vi "SPD.Overall Progress tracker.vi"(8 "Error In":errorcluster, 9 "Num of temps":i32, 10 "Current temprature index":i32, 11 "Slide in":refnum<vi>) -> (0 "Error Out":errorcluster, 3 "Slide out":refnum<vi>)   [LabVIEW 2018]
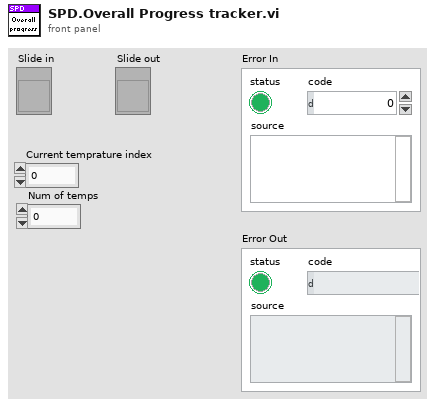
[diagram p1: front panel]
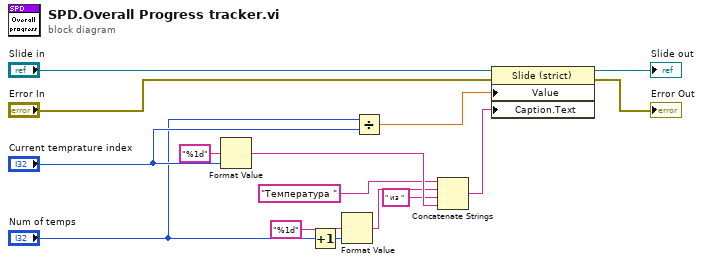
[diagram p0: block diagram]
diagram:
  n1 = Format Value(format string="%1d", value (0)="Current temprature index") -> (output string=w11:string)  [unwired: 1 in]
  n2 = Increment(x="Num of temps") -> (x+1=w13:i32)
  n3 = Format Value(format string="%1d", value (0)=w13) -> (output string=w9:string)  [unwired: 1 in]
  n4 = Divide(x="Num of temps", y="Current temprature index") -> (x/y=w3:dbl)
  n5 = Concatenate Strings("Температура " ("string"), w9, " из " ("string"), w11) -> (w12:string)
  n6 = property on="Property Node" class="Slide (strict)"(reference="Slide in", error in="Error In", "Value"=w3, "Caption.Text"=w12) -> (reference out=→"Slide out":refnum<vi>, error out=→"Error Out":errorcluster)
